vi "Versus.vi"(11 "DataIn":T1={"Quem Joga"="", "Tabuleiro"={"(0,0)"="", "(1,0)"="", "(0,1)"="", "(1,1)"="", "(2,0)"="", "(1,2)"="", "(2,2)"="", "(0,2)"="", "(2,1) "=""}, "GameOption"=enum."Multiplayer local", "Turno"=FALSE, "Player"="", "Player 1"="", "Player 2"="", "Dificuldade"=enum."Easy", "Table"=[], "Row"=0, "Aceitar Convite"=FALSE, "Inviter line"=0, "diretório"=path "", "Logout - panel close"=FALSE, "StartGame"=FALSE, "MatchData.lvclass"=refnum, "GameMode"=enum."Single Easy", "Level State"=FALSE}) -> (3 "DataOut":T1={"Quem Joga"="", "Tabuleiro"={"(0,0)"="", "(1,0)"="", "(0,1)"="", "(1,1)"="", "(2,0)"="", "(1,2)"="", "(2,2)"="", "(0,2)"="", "(2,1) "=""}, "GameOption"=enum."Multiplayer local", "Turno"=FALSE, "Player"="", "Player 1"="", "Player 2"="", "Dificuldade"=enum."Easy", "Table"=[], "Row"=0, "Aceitar Convite"=FALSE, "Inviter line"=0, "diretório"=path "", "Logout - panel close"=FALSE, "StartGame"=FALSE, "MatchData.lvclass"=refnum, "GameMode"=enum."Single Easy", "Level State"=FALSE})   [LabVIEW 2018]
doc: "SubVI criada para apagar a coluna de adversário na linha de quem convidou e de quem foi convidado no caso de recusa ou de fim de jogo"
uses:
  controls/DataIn.ctl
  MatchDataClasses/MatchData/MatchData.lvclass
  controls/Tabuleiro.ctl
  controls/Table.ctl
  <vilib>/Utility/file.llb/Write Delimited Spreadsheet (string).vi
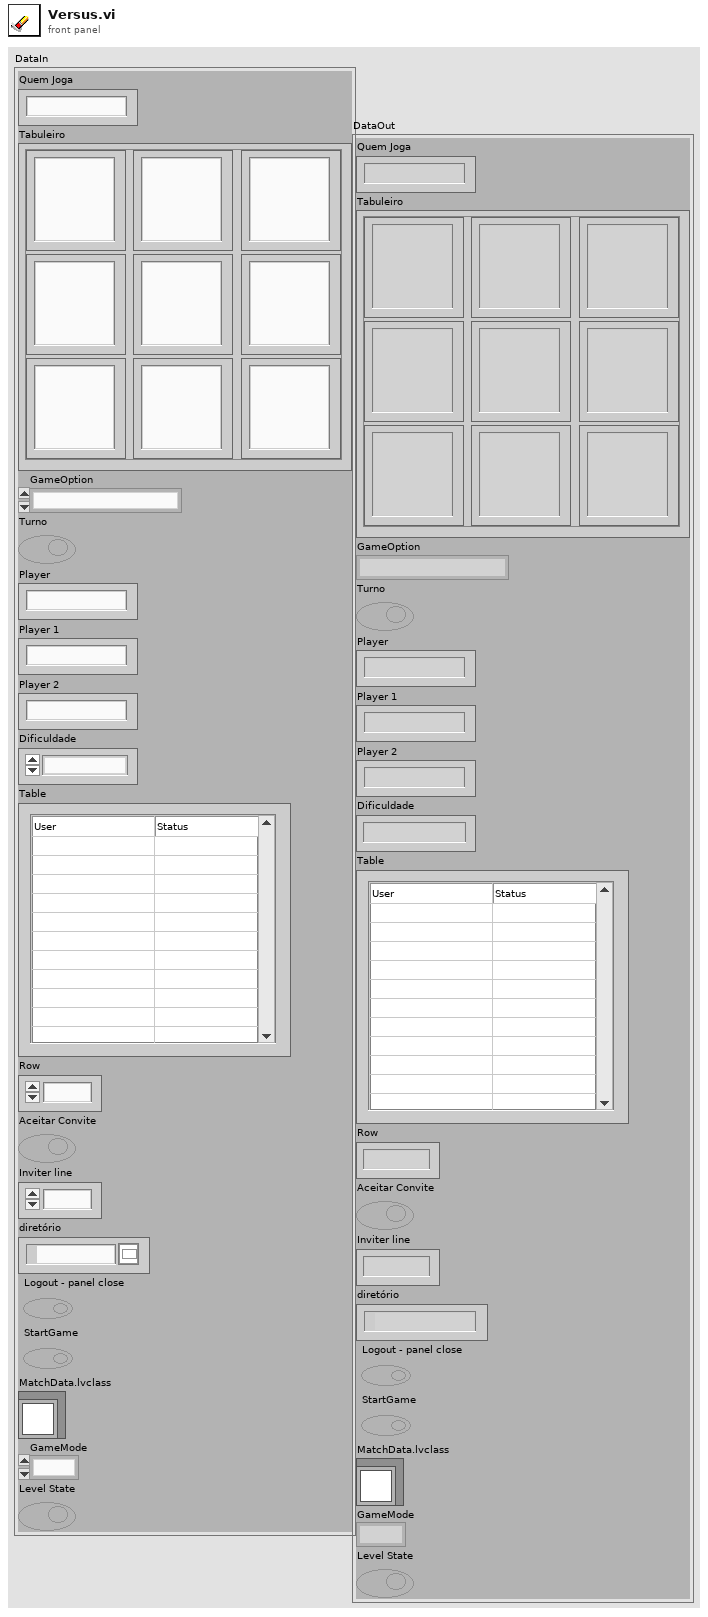
[diagram p1: front panel]
types:
  T1 = typedef "DataIn.ctl" = cluster{"Quem Joga":string, "Tabuleiro":T2, "GameOption":enum16{"Single Player", "Multiplayer local", "Multiplayer remoto", "Wait for Event", "Initialize", "Stop"}, "Turno":bool, "Player":string, "Player 1":string, "Player 2":string, "Dificuldade":enum16{"Easy", "Medium", "Hard"}, "Table":T3, "Row":u32, "Aceitar Convite":bool, "Inviter line":u32, "diretório":path, "Logout - panel close":bool, "StartGame":bool, "MatchData.lvclass":refnum<class "MatchData.lvclass">, "GameMode":enum16{"Single Easy", "Single Medium", "Single Hard", "Local", "Remote"}, "Level State":bool}
  T2 = typedef "Tabuleiro.ctl" = cluster{"(0,0)":string, "(1,0)":string, "(0,1)":string, "(1,1)":string, "(2,0)":string, "(1,2)":string, "(2,2)":string, "(0,2)":string, "(2,1) ":string}
  T3 = typedef "Table.ctl" = string[][]
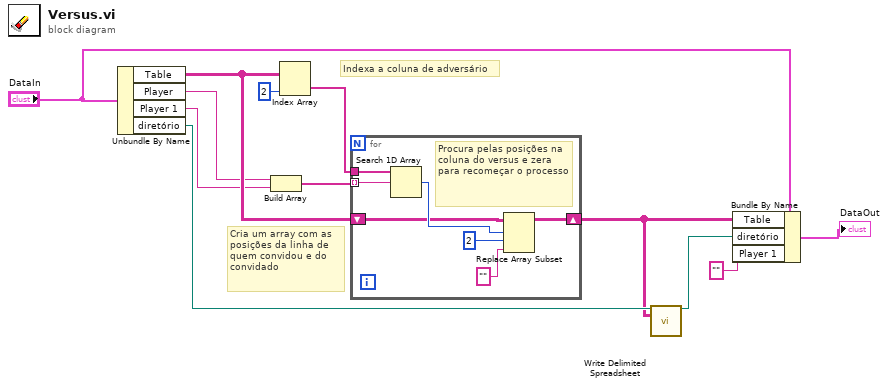
[diagram p0: block diagram]
diagram:
  # "Cria um array com as posições da linha de quem convidou e do convidado"
  # "Indexa a coluna de adversário"
  n1 = Unbundle By Name("DataIn") -> ("Table"=w8:T3, "Player"=w6:string, "Player 1"=w5:string, "diretório"=w4:path)
  n2 = Build Array(w6, w5) -> (w7:string[])
  n3 = Index Array(array=w8, index (col)=2 ("disabled index (col)")) -> (element=w10:string[])  [unwired: 1 in]
  n4 = for {
    tunnel: w7 -> [w13] mode=indexing
    tunnel: w10 -> [w16]
    shift-right: [w14] -> w2
    shift-left: w8 -> [w15]
    # "Procura pelas posições na coluna do versus e zera para recomeçar o processo"
    n5 = Search 1D Array(1D array=w16, element=w13) -> (index of element=w17:i32)  [unwired: 1 in]
    n6 = Replace Array Subset(array=w15, new element="", index (row)=w17, index (col)=2 ("disabled index (col)")) -> (w14:T3)
  }
  n7 = call-poly <vilib>:"Write Delimited Spreadsheet.vi"("file path (dialog if empty)"=w4, "2D data"=w2) -> ("new file path (Not A Path if cancelled)"=w3:path)  [unwired: 12 in, 1 out]
  n8 = Bundle By Name(cluster="DataIn", "Table"=w2, "diretório"=w3, "Player 1"="") -> (→"DataOut":T1)
